vi "mclb_move.vi"(7 "remove bevel (3px)":i32=3, 8 "Panel Resize.NewBnds":T1, 9 "FP.Origin":T4, 10 "FP.PanelBounds":T1, 11 "FP.WinBounds":T1) -> (2 "bounds":T2, 3 "pos":T3)   [LabVIEW 2017, in "rywindow.lvclass"]
uses:
  rywindow.lvclass
  <vilib>/Utility/miscctls.llb/LVPointTypeDef.ctl
  <vilib>/Utility/miscctls.llb/LVRectTypeDef.ctl
  <vilib>/Utility/miscctls.llb/LVPositionTypeDef.ctl
  <vilib>/Utility/miscctls.llb/LVBoundsTypeDef.ctl
panel:
  out "New.PanelSize":cluster{"Width":i16, "Height":i16}
  out "FP.MenuSize":cluster{"Width":i16, "Height":i16}
  out "FP.PanelSize":cluster{"Width":i16, "Height":i16}
  out "FP.WinSize":cluster{"Width":i16, "Height":i16}
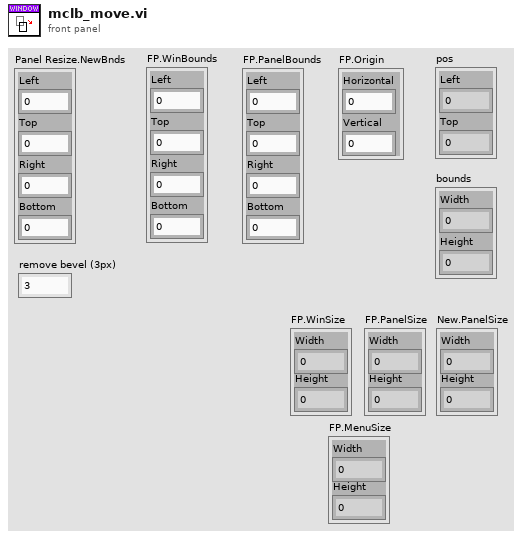
[diagram p1: front panel]
types:
  T1 = typedef "LVRectTypeDef.ctl" = cluster{"Left":i16, "Top":i16, "Right":i16, "Bottom":i16}
  T2 = typedef "LVBoundsTypeDef.ctl" = cluster{"Width":u32, "Height":u32}
  T3 = typedef "LVPositionTypeDef.ctl" = cluster{"Left":i32, "Top":i32}
  T4 = typedef "LVPointTypeDef.ctl" = cluster{"Horizontal":i16, "Vertical":i16}
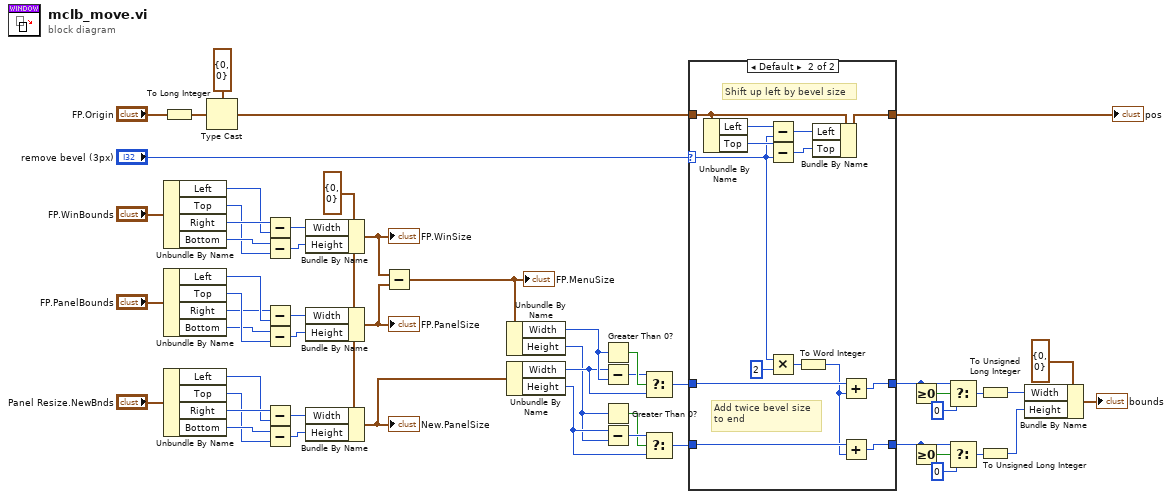
[diagram p0: block diagram]
diagram:
  w28 = cluster{"Width":i16, "Height":i16} {"Width"=0, "Height"=0} ("FP.WinSize")
  n1 = To Long Integer(number="FP.Origin") -> (32bit integer=w36:cluster{"Horizontal":i32, "Vertical":i32})
  n2 = Unbundle By Name("FP.WinBounds") -> ("Left"=w53:i16, "Top"=w51:i16, "Right"=w54:i16, "Bottom"=w52:i16)
  n3 = Unbundle By Name("FP.PanelBounds") -> ("Left"=w48:i16, "Top"=w50:i16, "Right"=w47:i16, "Bottom"=w49:i16)
  n4 = Unbundle By Name("Panel Resize.NewBnds") -> ("Left"=w44:i16, "Top"=w42:i16, "Right"=w45:i16, "Bottom"=w43:i16)
  n5 = Type Cast(type=T3 {"Left"=0, "Top"=0} ("pos 2"), x=w36) -> (*(type *) &x=w12:T3)
  n6 = Subtract(x=w54, y=w53) -> (x-y=w32:i16)
  n7 = Subtract(x=w52, y=w51) -> (x-y=w31:i16)
  n8 = Subtract(x=w47, y=w48) -> (x-y=w34:i16)
  n9 = Subtract(x=w49, y=w50) -> (x-y=w33:i16)
  n10 = Subtract(x=w45, y=w44) -> (x-y=w30:i16)
  n11 = Subtract(x=w43, y=w42) -> (x-y=w29:i16)
  n12 = Bundle By Name(cluster=w28, "Width"=w32, "Height"=w31) -> (w46:cluster{"Width":i16, "Height":i16})
  "FP.WinSize" <- w46
  n13 = Bundle By Name(cluster=w28, "Width"=w34, "Height"=w33) -> (w41:cluster{"Width":i16, "Height":i16})
  "FP.PanelSize" <- w41
  n14 = Bundle By Name(cluster=w28, "Width"=w30, "Height"=w29) -> (w26:cluster{"Width":i16, "Height":i16})
  "New.PanelSize" <- w26
  n15 = Subtract(x=w46, y=w41) -> (x-y=w27:cluster{"Width":i16, "Height":i16})
  "FP.MenuSize" <- w27
  n16 = Unbundle By Name(w27) -> ("Width"=w24:i16, "Height"=w18:i16)
  n17 = Unbundle By Name(w26) -> ("Width"=w22:i16, "Height"=w19:i16)
  n18 = Greater Than 0?(x=w24) -> (x > 0?=w25:bool)
  n19 = Subtract(x=w22, y=w24) -> (x-y=w23:i16)
  n20 = Greater Than 0?(x=w18) -> (x > 0?=w20:bool)
  n21 = Subtract(x=w19, y=w18) -> (x-y=w21:i16)
  n22 = Select(t=w23, s=w25, f=w22) -> (s? t:f=w17:i16)
  n23 = Select(t=w21, s=w20, f=w19) -> (s? t:f=w16:i16)
  n24 = case shown="Default" "remove bevel (3px)" {
    selector: "remove bevel (3px)" -> [_ w61]
    tunnel: w17 -> [w56 w71]
    tunnel: w16 -> [w55 w70]
    tunnel: w12 -> [w57 w69]
    tunnel: [w57 w68] -> w11
    tunnel: [w56 w63] -> w6
    tunnel: [w55 w62] -> w2
    frame 0 {
    }
    frame Default {
      # "Add twice bevel size\nto end"
      # "Shift up left by bevel size"
      n25 = Unbundle By Name(w69) -> ("Left"=w67:i32, "Top"=w65:i32)
      n26 = Subtract(x=w67, y=w61) -> (x-y=w66:i32)
      n27 = Subtract(x=w65, y=w61) -> (x-y=w64:i32)
      n28 = Multiply(x=w61, y=2) -> (x*y=w59:i32)
      n29 = To Word Integer(number=w59) -> (16bit integer=w58:i16)
      n30 = Bundle By Name(cluster=w69, "Left"=w66, "Top"=w64) -> (w68:T3)
      n31 = Add(x=w71, y=w58) -> (x+y=w63:i16)
      n32 = Add(x=w70, y=w58) -> (x+y=w62:i16)
    }
  }
  "pos" <- w11
  n33 = Greater Or Equal To 0?(x=w6) -> (x >= 0?=w8:bool)
  n34 = Greater Or Equal To 0?(x=w2) -> (x >= 0?=w3:bool)
  n35 = Select(t=w6, s=w8, f=i16 0) -> (s? t:f=w7:i16)
  n36 = Select(t=w2, s=w3, f=i16 0) -> (s? t:f=w1:i16)
  n37 = To Unsigned Long Integer(number=w7) -> (unsigned 32bit integer=w14:u32)
  n38 = To Unsigned Long Integer(number=w1) -> (unsigned 32bit integer=w13:u32)
  n39 = Bundle By Name(cluster=T2 {"Width"=0, "Height"=0} ("bounds"), "Width"=w14, "Height"=w13) -> (→"bounds":T2)
